vi "Lab Panel V5.20.vi"() -> ()   [LabVIEW 2013] (continued)
                n1788 = property on="O/I  LAB04-1" class="Bool (strict)"("DisabledEnum"=w3333) -> ()  [unwired: 2 in, 2 out]
                n1789 = property on="O/I  LAB04-2" class="Bool (strict)"("DisabledEnum"=w3332) -> ()  [unwired: 2 in, 2 out]
                n1790 = property on="O/I  LAB03-2" class="Bool (strict)"("DisabledEnum"=w3334) -> ()  [unwired: 2 in, 2 out]
                n1791 = Not(x=w3339) -> (.not. x?=w3340:bool)
                n1792 = Not(x=w3338) -> (.not. x?=w3341:bool)
                n1793 = Not(x=w3337) -> (.not. x?=w3342:bool)
                n1794 = property on="RESULT LAB05-2" class="Bool (strict)"("Visible"=w3340) -> ()  [unwired: 2 in, 2 out]
                n1795 = property on="RESULT LAB05-1" class="Bool (strict)"("Visible"=w3341) -> ()  [unwired: 2 in, 2 out]
                n1796 = Not(x=w3336) -> (.not. x?=w3343:bool)
                n1797 = property on="RESULT LAB04-2" class="Bool (strict)"("Visible"=w3342) -> ()  [unwired: 2 in, 2 out]
                n1798 = Not(x=w3335) -> (.not. x?=w3344:bool)
                n1799 = property on="RESULT LAB04-1" class="Bool (strict)"("Visible"=w3343) -> ()  [unwired: 2 in, 2 out]
                n1800 = property on="RESULT LAB03-2" class="Bool (strict)"("Visible"=w3344) -> ()  [unwired: 2 in, 2 out]
              }
              frame #2 {
                # "disable calibrate if any test running"
                n1801 = Or(x=w3367, y=w3366) -> (x .or. y?=w3360:bool)
                n1802 = Or(x=w3369, y=w3368) -> (x .or. y?=w3362:bool)
                n1803 = Or(x=w3373, y=w3372) -> (x .or. y?=w3364:bool)
                n1804 = Or(x=w3371, y=w3370) -> (x .or. y?=w3363:bool)
                n1805 = Or(x=w3375, y=w3374) -> (x .or. y?=w3365:bool)
                n1806 = Or(x=w3363, y=w3362) -> (x .or. y?=w3361:bool)
                n1807 = Or(x=w3365, y=w3364) -> (x .or. y?=w3359:bool)
                n1808 = Or(x=w3361, y=w3360) -> (x .or. y?=w3358:bool)
                n1809 = Or(x=w3359, y=w3358) -> (x .or. y?=w3357:bool)
                n1810 = case shown="False" w3357 {
                  tunnel: [0 2] -> w3356
                  frame False {
                  }
                  frame True {
                  }
                }
                n1811 = property on="JIG TEST" class="Clust (strict)"("DisabledEnum"=w3356) -> ()  [unwired: 2 in, 2 out]
                n1812 = property on="Network Directory" class="Path"("DisabledEnum"=w3356) -> ()  [unwired: 2 in, 2 out]
                n1813 = property on="MAIL SETTINGS" class="Clust (strict)"("DisabledEnum"=w3356) -> ()  [unwired: 2 in, 2 out]
                n1814 = property on="SET (cal)" class="Bool (strict)"("DisabledEnum"=w3356) -> ()  [unwired: 2 in, 2 out]
                n1815 = property on="ADMIN" class="Bool (strict)"("DisabledEnum"=0) -> ()  [unwired: 2 in, 2 out]
              }
            }
          }
          frame #8 {
            # "drive jigs"
            n1816 = stacked-sequence {
              frame #0 {
                # "jig on"
                n1817 = local read "jig cycle"() -> (w3383:dbl)
                n1818 = property on="JIG TEST" class="Clust (strict)"() -> ("DisabledEnum"=w3380:T16)  [unwired: 2 in, 2 out]
                n1819 = Equal?(x=w3380, y=2) -> (x = y?=w3379:bool)
                n1820 = Equal?(x=w3383, y=0) -> (x = y?=w3381:bool)
                n1821 = And(x=w3381, y=w3379) -> (x .and. y?=w3378:bool)
                n1822 = case shown="True" w3378 {
                  frame False {
                  }
                  frame True {
                    n1823 = local read "run lab01-1"() -> (w3394:bool)
                    n1824 = local read "run lab01-2"() -> (w3393:bool)
                    n1825 = local read "run lab02-1"() -> (w3392:bool)
                    n1826 = local read "run lab02-2"() -> (w3391:bool)
                    n1827 = local read "run lab03-1"() -> (w3390:bool)
                    n1828 = local read "run lab03-2"() -> (w3389:bool)
                    n1829 = local read "run lab04-1"() -> (w3388:bool)
                    n1830 = local read "run lab04-2"() -> (w3387:bool)
                    n1831 = local read "run lab05-1"() -> (w3386:bool)
                    n1832 = local read "run lab05-2"() -> (w3385:bool)
                    n1833 = local write "JIG LAB03-2"(w3389) -> ()
                    n1834 = local write "JIG LAB01-1"(w3394) -> ()
                    n1835 = local write "JIG LAB01-2"(w3393) -> ()
                    n1836 = local write "JIG LAB02-1"(w3392) -> ()
                    n1837 = local write "JIG LAB02-2"(w3391) -> ()
                    n1838 = local write "JIG LAB03-1"(w3390) -> ()
                    n1839 = local write "JIG LAB04-1"(w3388) -> ()
                    n1840 = local write "JIG LAB04-2"(w3387) -> ()
                    n1841 = local write "JIG LAB05-1"(w3386) -> ()
                    n1842 = local write "JIG LAB05-2"(w3385) -> ()
                  }
                }
              }
              frame #1 {
                # "jig off"
                n1843 = local read "jig cycle"() -> (w3401:dbl)
                n1844 = local read "on loops"() -> (w3400:dbl)
                n1845 = property on="JIG TEST" class="Clust (strict)"() -> ("DisabledEnum"=w3399:T16)  [unwired: 2 in, 2 out]
                n1846 = Equal?(x=w3399, y=2) -> (x = y?=w3397:bool)
                n1847 = Equal?(x=w3401, y=w3400) -> (x = y?=w3396:bool)
                n1848 = And(x=w3396, y=w3397) -> (x .and. y?=w3395:bool)
                n1849 = case shown="True" w3395 {
                  frame False {
                  }
                  frame True {
                    w3452 = FALSE
                    w3453 = TRUE
                    w3451 = 2
                    n1850 = local read "SELECT LAB05-2"() -> (w3442:T3)
                    n1851 = local read "SELECT LAB04-2"() -> (w3444:T3)
                    n1852 = local read "SELECT LAB04-1"() -> (w3445:T3)
                    n1853 = local read "SELECT LAB05-1"() -> (w3443:T3)
                    n1854 = local read "SELECT LAB03-2"() -> (w3446:T3)
                    n1855 = local read "SELECT LAB02-1"() -> (w3449:T3)
                    n1856 = local read "SELECT LAB03-1"() -> (w3447:T3)
                    n1857 = local read "SELECT LAB02-2"() -> (w3448:T3)
                    n1858 = local read "SELECT LAB01-2"() -> (w3450:T3)
                    n1859 = local read "run lab05-1"() -> (w3412:bool)
                    n1860 = local read "run lab05-2"() -> (w3411:bool)
                    n1861 = local read "run lab04-2"() -> (w3413:bool)
                    n1862 = local read "SELECT LAB01-1"() -> (w3454:T3)
                    n1863 = local read "run lab04-1"() -> (w3414:bool)
                    n1864 = local read "run lab01-1"() -> (w3430:bool)
                    n1865 = local read "run lab01-2"() -> (w3419:bool)
                    n1866 = local read "run lab03-2"() -> (w3415:bool)
                    n1867 = local read "run lab03-1"() -> (w3416:bool)
                    n1868 = local read "run lab02-1"() -> (w3418:bool)
                    n1869 = local read "run lab02-2"() -> (w3417:bool)
                    n1870 = Equal?(x=w3451, y=w3447) -> (x = y?=w3425:bool)
                    n1871 = Equal?(x=w3451, y=w3446) -> (x = y?=w3424:bool)
                    n1872 = Equal?(x=w3451, y=w3445) -> (x = y?=w3423:bool)
                    n1873 = Equal?(x=w3451, y=w3444) -> (x = y?=w3422:bool)
                    n1874 = Equal?(x=w3451, y=w3443) -> (x = y?=w3421:bool)
                    n1875 = Equal?(x=w3451, y=w3442) -> (x = y?=w3420:bool)
                    n1876 = Equal?(x=w3451, y=w3454) -> (x = y?=w3431:bool)
                    n1877 = Equal?(x=w3451, y=w3449) -> (x = y?=w3427:bool)
                    n1878 = Equal?(x=w3451, y=w3448) -> (x = y?=w3426:bool)
                    n1879 = Equal?(x=w3451, y=w3450) -> (x = y?=w3428:bool)
                    n1880 = And(x=w3422, y=w3413) -> (x .and. y?=w3404:bool)
                    n1881 = And(x=w3425, y=w3416) -> (x .and. y?=w3407:bool)
                    n1882 = And(x=w3423, y=w3414) -> (x .and. y?=w3405:bool)
                    n1883 = And(x=w3420, y=w3411) -> (x .and. y?=w3402:bool)
                    n1884 = And(x=w3426, y=w3417) -> (x .and. y?=w3408:bool)
                    n1885 = And(x=w3424, y=w3415) -> (x .and. y?=w3406:bool)
                    n1886 = And(x=w3421, y=w3412) -> (x .and. y?=w3403:bool)
                    n1887 = And(x=w3428, y=w3419) -> (x .and. y?=w3410:bool)
                    n1888 = And(x=w3431, y=w3430) -> (x .and. y?=w3429:bool)
                    n1889 = And(x=w3427, y=w3418) -> (x .and. y?=w3409:bool)
                    n1890 = Select(t=w3453, s=w3429, f=w3452) -> (s? t:f=w3432:bool)
                    n1891 = Select(t=w3453, s=w3410, f=w3452) -> (s? t:f=w3433:bool)
                    n1892 = Select(t=w3453, s=w3409, f=w3452) -> (s? t:f=w3434:bool)
                    n1893 = Select(t=w3453, s=w3408, f=w3452) -> (s? t:f=w3435:bool)
                    n1894 = Select(t=w3453, s=w3407, f=w3452) -> (s? t:f=w3436:bool)
                    n1895 = Select(t=w3453, s=w3406, f=w3452) -> (s? t:f=w3437:bool)
                    n1896 = Select(t=w3453, s=w3405, f=w3452) -> (s? t:f=w3438:bool)
                    n1897 = Select(t=w3453, s=w3404, f=w3452) -> (s? t:f=w3439:bool)
                    n1898 = Select(t=w3453, s=w3403, f=w3452) -> (s? t:f=w3440:bool)
                    n1899 = Select(t=w3453, s=w3402, f=w3452) -> (s? t:f=w3441:bool)
                    n1900 = local write "JIG LAB03-2"(w3437) -> ()
                    n1901 = local write "JIG LAB02-1"(w3434) -> ()
                    n1902 = local write "JIG LAB02-2"(w3435) -> ()
                    n1903 = local write "JIG LAB01-2"(w3433) -> ()
                    n1904 = local write "JIG LAB03-1"(w3436) -> ()
                    n1905 = local write "JIG LAB01-1"(w3432) -> ()
                    n1906 = local write "JIG LAB05-2"(w3441) -> ()
                    n1907 = local write "JIG LAB04-1"(w3438) -> ()
                    n1908 = local write "JIG LAB05-1"(w3440) -> ()
                    n1909 = local write "JIG LAB04-2"(w3439) -> ()
                  }
                }
              }
            }
          }
          frame #9 {
            # "enable  jig test output if no test busy"
            n1910 = property on="JIG TEST" class="Clust (strict)"() -> ("DisabledEnum"=w3457:T16)  [unwired: 2 in, 2 out]
            n1911 = Equal?(x=w3457, y=0) -> (x = y?=w3455:bool)
            n1912 = case shown="True" w3455 {
              frame False {
              }
              frame True {
                n1913 = local read "JIG TEST"() -> (w3468:T10)
                n1914 = Unbundle(w3468) -> ("LAB01-1"=w3467:bool, "LAB01-2"=w3466:bool, "LAB02-1"=w3465:bool, "LAB02-2"=w3464:bool, "LAB03-1"=w3463:bool, "LAB03-2"=w3462:bool, "LAB04-1"=w3461:bool, "LAB04-2"=w3460:bool, "LAB05-1"=w3459:bool, "LAB05-2"=w3458:bool)
                n1915 = local write "JIG LAB05-1"(w3459) -> ()
                n1916 = local write "JIG LAB05-2"(w3458) -> ()
                n1917 = local write "JIG LAB04-1"(w3461) -> ()
                n1918 = local write "JIG LAB04-2"(w3460) -> ()
                n1919 = local write "JIG LAB03-2"(w3462) -> ()
                n1920 = local write "JIG LAB01-1"(w3467) -> ()
                n1921 = local write "JIG LAB02-1"(w3465) -> ()
                n1922 = local write "JIG LAB03-1"(w3463) -> ()
                n1923 = local write "JIG LAB01-2"(w3466) -> ()
                n1924 = local write "JIG LAB02-2"(w3464) -> ()
              }
            }
          }
          frame #10 {
            # "Drive digital output and reset USB and temperature network if required."
            n1925 = global read "Global display 3.vi" "cycle O/F"() -> (w3478:bool)
            n1926 = local read "O/I  LAB05-2"() -> (w3471:bool)
            n1927 = local read "O/I  LAB05-1"() -> (w3473:bool)
            n1928 = local read "JIG LAB05-2"() -> (w3470:bool)
            n1929 = local read "O/I  LAB04-2"() -> (w3475:bool)
            n1930 = local read "JIG LAB05-1"() -> (w3472:bool)
            n1931 = local read "JIG LAB04-2"() -> (w3474:bool)
            n1932 = local read "O/I  LAB03-1"() -> (w3489:bool)
            n1933 = local read "O/I  LAB04-1"() -> (w3485:bool)
            n1934 = local read "O/I  LAB02-1"() -> (w3493:bool)
            n1935 = local read "O/I  LAB02-2"() -> (w3491:bool)
            n1936 = local read "O/I  LAB03-2"() -> (w3487:bool)
            n1937 = local read "JIG LAB04-1"() -> (w3484:bool)
            n1938 = local read "JIG LAB03-2"() -> (w3486:bool)
            n1939 = local read "O/I  LAB01-2"() -> (w3495:bool)
            n1940 = local read "JIG LAB02-1"() -> (w3492:bool)
            n1941 = local read "JIG LAB02-2"() -> (w3490:bool)
            n1942 = local read "JIG LAB03-1"() -> (w3488:bool)
            n1943 = local read "O/I  LAB01-1"() -> (w3497:bool)
            n1944 = local read "JIG LAB01-2"() -> (w3494:bool)
            n1945 = local read "JIG LAB01-1"() -> (w3496:bool)
            n1946 = case shown="False" w3478 {
              tunnel: [w3578 FALSE] -> w3477
              frame False {
                n1947 = local read "Analog error"() -> (w3577:bool)
                n1948 = local read "Reset Measuring"() -> (w3576:bool)
                n1949 = Or(x=w3576, y=w3577) -> (x .or. y?=w3578:bool)
              }
              frame True {
              }
            }
            n1950 = Build Array(w3490, w3489, w3488, w3487, w3486, w3485, w3484) -> (w3482:bool[])
            n1951 = Build Array(w3497, w3496, w3495, w3494, w3493, w3492, w3491) -> (w3483:bool[])
            n1952 = Build Array(w3475, w3474, w3473, w3472, w3471, w3470, FALSE) -> (w3481:bool[])
            n1953 = Not(x=w3478) -> (.not. x?=w3479:bool)
            n1954 = local read "Simulate"() -> (w3480:bool)
            n1955 = And(x=w3479, y=w3477) -> (x .and. y?=w3476:bool)
            n1956 = stacked-sequence {
              tunnel: w3483 -> [w3501 w3507]
              tunnel: w3482 -> [w3500 w3506]
              tunnel: w3481 -> [w3499 w3505]
              tunnel: w3480 -> [w3498 w3508]
              tunnel: w3476 -> [_ w3509]
              frame #0 {
                # "drive outputs for normal use"
                n1957 = case shown="False" w3498 {
                  tunnel: w3501 -> [w3504 _]
                  tunnel: w3500 -> [w3503 _]
                  tunnel: w3499 -> [w3502 _]
                  frame False {
                    n1958 = call "sub vi - Drive Relays All v6.vi"("Array #2"=w3502, "Array #1"=w3503, "Array #0"=w3504) -> ()  [unwired: 8 in, 1 out]
                  }
                  frame True {
                  }
                }
              }
              frame #1 {
                # "system reset routine"
                n1959 = case shown="True" w3509 {
                  tunnel: w3508 -> [_ w3513]
                  tunnel: w3507 -> [_ w3512]
                  tunnel: w3506 -> [_ w3511]
                  tunnel: w3505 -> [_ w3510]
                  frame False {
                  }
                  frame True {
                    n1960 = stacked-sequence {
                      seq-local: [w3515 _ _] -> [_ w3521 _]
                      tunnel: w3513 -> [_ w3525 _]
                      tunnel: w3512 -> [_ w3524 _]
                      tunnel: w3511 -> [_ w3523 _]
                      tunnel: w3510 -> [_ w3522 _]
                      frame #0 {
                        n1961 = case shown="False" "Auto Reset" {
                          tunnel: [w3518 FALSE] -> w3516
                          frame False {
                            n1962 = Two Button Dialog(message="System reset") -> (T button?=w3518:bool)  [unwired: 2 in]
                          }
                          frame True {
                          }
                        }
                        n1963 = local write "Tab Control 2"(5) -> ()
                        n1964 = Or(x="Auto Reset", y=w3516) -> (x .or. y?=w3515:bool)
                      }
                      frame #1 {
                        n1965 = case shown="True" w3521 {
                          tunnel: w3525 -> [_ w3531]
                          tunnel: w3524 -> [_ w3530]
                          tunnel: w3523 -> [_ w3529]
                          tunnel: w3522 -> [_ w3528]
                          frame False {
                          }
                          frame True {
                            n1966 = stacked-sequence {
                              tunnel: w3531 -> [_ w3549 _]
                              tunnel: bool[] [] -> [w3534 w3548 w3557]
                              tunnel: w3530 -> [_ _ w3556]
                              tunnel: w3529 -> [w3533 _ w3555]
                              tunnel: w3528 -> [w3532 _ w3554]
                              tunnel: 3000 -> [w3535 _ w3553]
                              frame #0 {
                                # "switch off test stations for system reset"
                                n1967 = stacked-sequence {
                                tunnel: w3535 -> [w3539 w3543 w3545]
                                tunnel: w3534 -> [w3538 w3542 w3546]
                                tunnel: w3533 -> [w3537 _ _]
                                tunnel: w3532 -> [w3536 w3541 _]
                                frame #0 {
                                # "drive 1st 7 inputs"
                                n1968 = call "sub vi - Drive Relays All v6.vi"("Array #2"=w3536, "Array #1"=w3537, "Array #0"=w3538) -> ()  [unwired: 8 in, 1 out]
                                n1969 = call "Message Display V1.vi"("Message"="Delay off LAB 01-1 to 02-1", "Delay mS"=w3539) -> ()  [unwired: 10 in]
                                }
                                frame #1 {
                                # "drive 2nd 7 inputs"
                                n1970 = call "sub vi - Drive Relays All v6.vi"("Array #2"=w3541, "Array #1"=w3542, "Array #0"=w3542) -> ()  [unwired: 8 in, 1 out]
                                n1971 = call "Message Display V1.vi"("Message"="Delay off LAB 02-2 to 04-1", "Delay mS"=w3543) -> ()  [unwired: 10 in]
                                }
                                frame #2 {
                                # "drive 3rd 7 inputs"
                                n1972 = call "sub vi - Drive Relays All v6.vi"("Array #2"=w3546, "Array #1"=w3546, "Array #0"=w3546) -> ()  [unwired: 8 in, 1 out]
                                n1973 = call "Message Display V1.vi"("Message"="Delay off LAB 04-2 to 05-2", "Delay mS"=w3545) -> ()  [unwired: 10 in]
                                }
                                }
                              }
                              frame #1 {
                                # "reset all usb modules"
                                n1974 = stacked-sequence {
                                tunnel: w3549 -> [_ w3552]
                                tunnel: w3548 -> [w3551 _]
                                frame #0 {
                                n1975 = call "sub vi - Drive Relays All v6.vi"("Array #2"=bool[] [FALSE, FALSE, FALSE, FALSE, FALSE, FALSE, TRUE], "Array #1"=w3551, "Array #0"=w3551) -> ()  [unwired: 8 in, 1 out]
                                }
                                frame #1 {
                                n1976 = call "Reset Meas v 4.vi"("simulate"=w3552) -> ()  [unwired: 11 in]
                                }
                                }
                              }
                              frame #2 {
                                # "switch test stations back on after reset"
                                n1977 = stacked-sequence {
                                tunnel: w3557 -> [w3561 w3564 _]
                                tunnel: w3556 -> [w3560 w3566 w3571]
                                tunnel: w3553 -> [w3559 w3562 w3568]
                                tunnel: w3555 -> [_ w3565 w3570]
                                tunnel: w3554 -> [_ _ w3567]
                                frame #0 {
                                # "drive 1st 7 inputs"
                                n1978 = call "sub vi - Drive Relays All v6.vi"("Array #2"=w3561, "Array #1"=w3561, "Array #0"=w3560) -> ()  [unwired: 8 in, 1 out]
                                n1979 = call "Message Display V1.vi"("Message"="Delay on LAB 01-1 to 02-1", "Delay mS"=w3559) -> ()  [unwired: 10 in]
                                }
                                frame #1 {
                                # "drive 1st & 2nd outputs"
                                n1980 = call "sub vi - Drive Relays All v6.vi"("Array #2"=w3564, "Array #1"=w3565, "Array #0"=w3566) -> ()  [unwired: 8 in, 1 out]
                                n1981 = call "Message Display V1.vi"("Message"="Delay on LAB 02-2 to 04-1", "Delay mS"=w3562) -> ()  [unwired: 10 in]
                                }
                                frame #2 {
                                n1982 = call "sub vi - Drive Relays All v6.vi"("Array #2"=w3567, "Array #1"=w3570, "Array #0"=w3571) -> ()  [unwired: 8 in, 1 out]
                                n1983 = call "Message Display V1.vi"("Message"="Delay on LAB 04-2 to 05-2", "Delay mS"=w3568) -> ()  [unwired: 10 in]
                                }
                                }
                              }
                            }
                          }
                        }
                      }
                      frame #2 {
                        w3574 = 0
                        w3575 = FALSE
                        # "set all back to zero"
                        n1984 = local read "Resets Done"() -> (w3573:dbl)
                        n1985 = local write "Reset Measuring"(w3575) -> ()
                        n1986 = local write "Analog error"(w3575) -> ()
                        n1987 = local write "Error USB #0"(w3575) -> ()
                        n1988 = local write "Error USB #1"(w3575) -> ()
                        n1989 = local write "Error USB #2"(w3575) -> ()
                        n1990 = local write "Er USB#0"(w3574) -> ()
                        n1991 = local write "Er USB#1"(w3574) -> ()
                        n1992 = local write "Er USB#2"(w3574) -> ()
                        n1993 = Increment(x=w3573) -> (x+1=→"Resets Done":dbl)
                      }
                    }
                  }
                }
              }
            }
          }
          frame #11 {
            # "get all analog values from USB devices"
            n1994 = local read "on loops"() -> (w3586:dbl)
            n1995 = local read "jig cycle"() -> (w3583:dbl)
            n1996 = Add(x=w3586, y=1) -> (x+y=w3584:dbl)
            n1997 = Equal?(x=w3583, y=1) -> (x = y?=w3580:bool)
            n1998 = Equal?(x=w3583, y=w3584) -> (x = y?=w3582:bool)
            n1999 = Or(x=w3580, y=w3582) -> (x .or. y?=w3581:bool)
            n2000 = global write "Global display 3.vi" "cycle O/F"(w3580) -> ()
            n2001 = case shown="True" w3581 {
              tunnel: w3580 -> [_ w3590]
              frame False {
              }
              frame True {
                n2002 = local read "Simulate"() -> (w3593:bool)
                n2003 = case shown="False" w3593 {
                  tunnel: [w3609 0.3 ("Analog loop time")] -> w3600
                  tunnel: [w3608 dynamicdata[] [] ("array GRAPH")] -> w3599
                  tunnel: [w3607 w3614] -> w3598
                  tunnel: [w3606 w3614] -> w3597
                  tunnel: [w3605 w3614] -> w3596
                  tunnel: [w3604 w3614] -> w3595
                  tunnel: [w3603 w3614] -> w3594
                  tunnel: w3590 -> [_ w3618]
                  tunnel: [w3602 "Ambient Volts"] -> w3589
                  tunnel: [w3601 bool[] []] -> w3588
                  frame False {
                    n2004 = call "sub vi - Read Analog All v9.3.vi"() -> ("Analog loop time"=w3609:dbl, "array GRAPH"=w3608:dynamicdata[], "LAB01"=w3607:T26, "LAB02"=w3606:T27, "LAB03"=w3605:T28, "LAB04"=w3604:T29, "deg C"=w3602:dbl, "USB Error"=w3601:bool[], "LAB05"=w3603:T30)  [unwired: 7 in]
                  }
                  frame True {
                    n2005 = local read "ON amps"() -> (w3612:dbl)
                    n2006 = local read "OFF amps"() -> (w3613:dbl)
                    n2007 = local read "VOLTS"() -> (w3616:dbl)
                    n2008 = local read "PF"() -> (w3615:dbl)
                    n2009 = Select(t=w3612, s=w3618, f=w3613) -> (s? t:f=w3617:dbl)
                    n2010 = Bundle("OFF amps"=w3617, "VOLTS"=w3616, "PF"=w3615, "OFF amps"=w3617, "VOLTS"=w3616, "PF"=w3615) -> (w3614:T31)  [unwired: 1 in]
                  }
                }
                n2011 = local read "Simulate"() -> (w3592:bool)
                n2012 = stacked-sequence {
                  seq-local: [w3623 _ _ _ _ _ _ _] -> [_ _ _ _ _ _ _ _]
                  seq-local: [w3622 _ _ _ _ _ _ _] -> [_ _ _ _ _ _ _ _]
                  seq-local: [w3621 _ _ _ _ _ _ _] -> [_ _ _ _ _ _ _ w3818]
                  tunnel: w3600 -> [_ w3676 _ _ _ _ _ _]
                  tunnel: w3599 -> [_ w3673 _ _ _ _ _ _]
                  tunnel: w3598 -> [_ _ w3703 _ _ _ _ _]
                  tunnel: w3597 -> [_ _ _ w3731 _ _ _ _]
                  tunnel: w3596 -> [_ _ _ _ w3759 _ _ _]
                  tunnel: w3595 -> [_ _ _ _ _ w3787 _ _]
                  tunnel: w3594 -> [_ _ _ _ _ _ w3815 _]
                  tunnel: w3592 -> [_ _ w3702 w3730 w3758 w3786 w3814 w3820]
                  tunnel: T14 {"1  (A) cal"=1.0, "1 (V) cal"=1.0, "1 (PF) cal"=1.0, "1 (TL) cal"=1.0, "1 (TN) cal"=1.0, "2 (A) cal"=1.0, "2 (V) cal"=1.0, "2 (PF) cal"=1.0, "2 (TL) cal"=1.0, "2 (TN) cal"=1.0} ("CAL LAB01") -> [_ _ w3701 w3729 w3757 w3785 w3813 _]
                  tunnel: w3589 -> [_ _ _ _ _ _ _ w3819]
                  tunnel: w3588 -> [w3626 _ _ _ _ _ _ _]
                  frame #0 {
                    n2013 = Index Array(array=w3626, index=2) -> (element=w3621:bool)
                    n2014 = Index Array(array=w3626, index=1) -> (element=w3622:bool)
                    n2015 = Index Array(array=w3626, index=0) -> (element=w3623:bool)
                    n2016 = local write "Error USB #2"(w3621) -> ()
                    n2017 = local write "Error USB #0"(w3623) -> ()
                    n2018 = local write "Error USB #1"(w3622) -> ()
                    n2019 = stacked-sequence {
                      tunnel: w3623 -> [w3630 _ _ _]
                      tunnel: w3622 -> [_ w3635 _ _]
                      tunnel: 0 -> [w3629 w3634 w3639 _]
                      tunnel: w3621 -> [_ _ w3640 _]
                      frame #0 {
                        n2020 = case shown="True" w3630 {
                          tunnel: w3629 -> [w3631 _]
                          frame False {
                            n2021 = local write "Er USB#0"(w3631) -> ()
                          }
                          frame True {
                            n2022 = local read "Er USB#0"() -> (w3633:dbl)
                            n2023 = Increment(x=w3633) -> (x+1=→"Er USB#0":dbl)
                          }
                        }
                      }
                      frame #1 {
                        n2024 = case shown="True" w3635 {
                          tunnel: w3634 -> [w3636 _]
                          frame False {
                            n2025 = local write "Er USB#1"(w3636) -> ()
                          }
                          frame True {
                            n2026 = local read "Er USB#1"() -> (w3638:dbl)
                            n2027 = Increment(x=w3638) -> (x+1=→"Er USB#1":dbl)
                          }
                        }
                      }
                      frame #2 {
                        n2028 = case shown="True" w3640 {
                          tunnel: w3639 -> [w3641 _]
                          frame False {
                            n2029 = local write "Er USB#2"(w3641) -> ()
                          }
                          frame True {
                            n2030 = local read "Er USB#2"() -> (w3643:dbl)
                            n2031 = Increment(x=w3643) -> (x+1=→"Er USB#2":dbl)
                          }
                        }
                      }
                      frame #3 {
                        w3649 = 5
                        n2032 = local read "Er USB#2"() -> (w3650:dbl)
                        n2033 = local read "Er USB#0"() -> (w3652:dbl)
                        n2034 = local read "Er USB#1"() -> (w3651:dbl)
                        n2035 = Greater Or Equal?(x=w3652, y=w3649) -> (x >= y?=w3647:bool)
                        n2036 = Greater Or Equal?(x=w3651, y=w3649) -> (x >= y?=w3646:bool)
                        n2037 = Greater Or Equal?(x=w3650, y=w3649) -> (x >= y?=w3645:bool)
                        n2038 = Or(x=w3647, y=w3646) -> (x .or. y?=w3648:bool)
                        n2039 = Or(x=w3648, y=w3645) -> (x .or. y?=→"Analog error":bool)
                      }
                    }
                  }
                  frame #1 {
                    # "display graph data on ADM page"
                    n2040 = local write "AI"(TRUE) -> ()
                    n2041 = global write "Global 1.vi" "RATE(Hz)"("RATE (Hz)") -> ()
                    n2042 = global write "Global 1.vi" "SAMPLES"("SAMPLES") -> ()
                    n2043 = Index Array(array=w3673, index=6) -> (element=→"LAB04-1 (GRAPH)":dynamicdata)
                    n2044 = Index Array(array=w3673, index=7) -> (element=→"LAB04-2 (GRAPH)":dynamicdata)
                    n2045 = Index Array(array=w3673, index=9) -> (element=→"LAB05-2 (GRAPH)":dynamicdata)
                    n2046 = Index Array(array=w3673, index=8) -> (element=→"LAB05-1 (GRAPH)":dynamicdata)
                    n2047 = Index Array(array=w3673, index=5) -> (element=→"LAB03-2 (GRAPH)":dynamicdata)
                    n2048 = Index Array(array=w3673, index=0) -> (element=→"LAB01-1 (GRAPH)":dynamicdata)
                    n2049 = Index Array(array=w3673, index=1) -> (element=→"LAB01-2 (GRAPH)":dynamicdata)
                    n2050 = Index Array(array=w3673, index=2) -> (element=→"LAB02-1 (GRAPH)":dynamicdata)
                    n2051 = Index Array(array=w3673, index=3) -> (element=→"LAB02-2 (GRAPH)":dynamicdata)
                    n2052 = Index Array(array=w3673, index=4) -> (element=→"LAB03-1 (GRAPH)":dynamicdata)
                    "AI loop time" <- w3676
                  }
                  frame #2 {
                    n2053 = case shown="False" w3702 {
                      tunnel: [w3704 w3705] -> w3700
                      tunnel: w3701 -> [_ w3705]
                      frame False {
                        n2054 = local read "CAL LAB01"() -> (w3704:T14)
                      }
                      frame True {
                      }
                    }
                    n2055 = Unbundle By Name(w3703) -> ("OFF amps"=w3699:dbl, "VOLTS"=w3698:dbl, "PF"=w3697:dbl, "OFF amps"=w3696:dbl, "VOLTS"=w3695:dbl, "PF"=w3694:dbl)
                    n2056 = Unbundle By Name(w3700) -> ("1  (A) cal"=w3693:dbl, "1 (V) cal"=w3692:dbl, "1 (PF) cal"=w3691:dbl, "2 (A) cal"=w3690:dbl, "2 (V) cal"=w3689:dbl, "2 (PF) cal"=w3688:dbl)  [unwired: 4 out]
                    n2057 = Multiply(x=w3699, y=w3693) -> (x*y=w3686:dbl)
                    n2058 = Multiply(x=w3698, y=w3692) -> (x*y=w3685:dbl)
                    n2059 = Multiply(x=w3697, y=w3691) -> (x*y=w3684:dbl)
                    n2060 = Multiply(x=w3696, y=w3690) -> (x*y=w3682:dbl)
                    n2061 = Multiply(x=w3695, y=w3689) -> (x*y=w3681:dbl)
                    n2062 = Multiply(x=w3694, y=w3688) -> (x*y=w3680:dbl)
                    n2063 = local read "SIG LAB01-1"() -> (w3687:T2)
                    n2064 = local read "SIG LAB01-2"() -> (w3683:T2)
                    n2065 = Bundle By Name(cluster=w3687, "AMPS"=w3686, "VOLTS"=w3685, "PF"=w3684) -> (w3679:T2)
                    n2066 = Bundle By Name(cluster=w3683, "AMPS"=w3682, "VOLTS"=w3681, "PF"=w3680) -> (w3678:T2)
                    n2067 = global write "Global display 1.vi" "SIG LAB01-2"(w3678) -> ()
                    n2068 = global write "Global display 1.vi" "SIG LAB01-1"(w3679) -> ()
                    n2069 = local write "SIG LAB01-2"(w3678) -> ()
                    n2070 = local write "SIG LAB01-1"(w3679) -> ()
                  }
                  frame #3 {
                    n2071 = Unbundle By Name(w3731) -> ("OFF amps"=w3727:dbl, "VOLTS"=w3726:dbl, "PF"=w3725:dbl, "OFF amps"=w3724:dbl, "VOLTS"=w3723:dbl, "PF"=w3722:dbl)
                    n2072 = case shown="True" w3730 {
                      tunnel: [w3732 w3733] -> w3728
                      tunnel: w3729 -> [_ w3733]
                      frame False {
                        n2073 = local read "CAL LAB02"() -> (w3732:T15)
                      }
                      frame True {
                      }
                    }
                    n2074 = Unbundle By Name(w3728) -> ("1  (A) cal"=w3721:dbl, "1 (V) cal"=w3720:dbl, "1 (PF) cal"=w3719:dbl, "2 (A) cal"=w3718:dbl, "2 (V) cal"=w3717:dbl, "2 (PF) cal"=w3716:dbl)  [unwired: 4 out]
                    n2075 = Multiply(x=w3727, y=w3721) -> (x*y=w3714:dbl)
                    n2076 = Multiply(x=w3726, y=w3720) -> (x*y=w3713:dbl)
                    n2077 = Multiply(x=w3725, y=w3719) -> (x*y=w3712:dbl)
                    n2078 = Multiply(x=w3724, y=w3718) -> (x*y=w3710:dbl)
                    n2079 = Multiply(x=w3723, y=w3717) -> (x*y=w3709:dbl)
                    n2080 = Multiply(x=w3722, y=w3716) -> (x*y=w3708:dbl)
                    n2081 = local read "SIG LAB02-1"() -> (w3715:T2)
                    n2082 = local read "SIG LAB02-2"() -> (w3711:T2)
                    n2083 = Bundle By Name(cluster=w3715, "AMPS"=w3714, "VOLTS"=w3713, "PF"=w3712) -> (w3707:T2)
                    n2084 = Bundle By Name(cluster=w3711, "AMPS"=w3710, "VOLTS"=w3709, "PF"=w3708) -> (w3706:T2)
                    n2085 = global write "Global display 1.vi" "SIG LAB02-1"(w3707) -> ()
                    n2086 = local write "SIG LAB02-2"(w3706) -> ()
                    n2087 = global write "Global display 1.vi" "SIG LAB02-2"(w3706) -> ()
                    n2088 = local write "SIG LAB02-1"(w3707) -> ()
                  }
                  frame #4 {
                    n2089 = Unbundle By Name(w3759) -> ("OFF amps"=w3755:dbl, "VOLTS"=w3754:dbl, "PF"=w3753:dbl, "OFF amps"=w3752:dbl, "VOLTS"=w3751:dbl, "PF"=w3750:dbl)
                    n2090 = case shown="True" w3758 {
                      tunnel: [w3760 w3761] -> w3756
                      tunnel: w3757 -> [_ w3761]
                      frame False {
                        n2091 = local read "CAL LAB03"() -> (w3760:T14)
                      }
                      frame True {
                      }
                    }
                    n2092 = Unbundle By Name(w3756) -> ("1  (A) cal"=w3749:dbl, "1 (V) cal"=w3748:dbl, "1 (PF) cal"=w3747:dbl, "2 (A) cal"=w3746:dbl, "2 (V) cal"=w3745:dbl, "2 (PF) cal"=w3744:dbl)  [unwired: 4 out]
                    n2093 = Multiply(x=w3755, y=w3749) -> (x*y=w3742:dbl)
                    n2094 = Multiply(x=w3754, y=w3748) -> (x*y=w3736:dbl)
                    n2095 = Multiply(x=w3753, y=w3747) -> (x*y=w3741:dbl)
                    n2096 = Multiply(x=w3752, y=w3746) -> (x*y=w3739:dbl)
                    n2097 = Multiply(x=w3751, y=w3745) -> (x*y=w3738:dbl)
                    n2098 = Multiply(x=w3750, y=w3744) -> (x*y=w3737:dbl)
                    n2099 = local read "SIG LAB03-1"() -> (w3743:T2)
                    n2100 = local read "SIG LAB03-2"() -> (w3740:T2)
                    n2101 = Bundle By Name(cluster=w3743, "AMPS"=w3742, "VOLTS"=w3736, "PF"=w3741) -> (w3735:T2)
                    n2102 = Bundle By Name(cluster=w3740, "AMPS"=w3739, "VOLTS"=w3738, "PF"=w3737) -> (w3734:T2)
                    n2103 = global write "Global display 1.vi" "SIG LAB03-1"(w3735) -> ()
                    n2104 = global write "Global display 1.vi" "SIG LAB03-2"(w3734) -> ()
                    n2105 = local write "SIG LAB03-2"(w3734) -> ()
                    n2106 = local write "SIG LAB03-1"(w3735) -> ()
                  }
                  frame #5 {
                    n2107 = case shown="False" w3786 {
                      tunnel: [w3788 w3789] -> w3784
                      tunnel: w3785 -> [_ w3789]
                      frame False {
                        n2108 = local read "CAL LAB04"() -> (w3788:T14)
                      }
                      frame True {
                      }
                    }
                    n2109 = Unbundle By Name(w3787) -> ("OFF amps"=w3783:dbl, "VOLTS"=w3782:dbl, "PF"=w3781:dbl, "OFF amps"=w3780:dbl, "VOLTS"=w3779:dbl, "PF"=w3778:dbl)
                    n2110 = Unbundle By Name(w3784) -> ("1  (A) cal"=w3777:dbl, "1 (V) cal"=w3776:dbl, "1 (PF) cal"=w3775:dbl, "2 (A) cal"=w3774:dbl, "2 (V) cal"=w3773:dbl, "2 (PF) cal"=w3772:dbl)  [unwired: 4 out]
                    n2111 = Multiply(x=w3783, y=w3777) -> (x*y=w3770:dbl)
                    n2112 = Multiply(x=w3782, y=w3776) -> (x*y=w3769:dbl)
                    n2113 = Multiply(x=w3781, y=w3775) -> (x*y=w3768:dbl)
                    n2114 = Multiply(x=w3780, y=w3774) -> (x*y=w3766:dbl)
                    n2115 = Multiply(x=w3779, y=w3773) -> (x*y=w3765:dbl)
                    n2116 = Multiply(x=w3778, y=w3772) -> (x*y=w3764:dbl)
                    n2117 = local read "SIG LAB04-1"() -> (w3771:T2)
                    n2118 = local read "SIG LAB04-2"() -> (w3767:T2)
                    n2119 = Bundle By Name(cluster=w3771, "AMPS"=w3770, "VOLTS"=w3769, "PF"=w3768) -> (w3763:T2)
                    n2120 = Bundle By Name(cluster=w3767, "AMPS"=w3766, "VOLTS"=w3765, "PF"=w3764) -> (w3762:T2)
                    n2121 = global write "Global display 1.vi" "SIG LAB04-2"(w3762) -> ()
                    n2122 = global write "Global display 1.vi" "SIG LAB04-1"(w3763) -> ()
                    n2123 = local write "SIG LAB04-2"(w3762) -> ()
                    n2124 = local write "SIG LAB04-1"(w3763) -> ()
                  }
                  frame #6 {
                    n2125 = Unbundle By Name(w3815) -> ("OFF amps"=w3811:dbl, "VOLTS"=w3792:dbl, "PF"=w3810:dbl, "OFF amps"=w3809:dbl, "VOLTS"=w3808:dbl, "PF"=w3807:dbl)
                    n2126 = case shown="False" w3814 {
                      tunnel: [w3816 w3817] -> w3812
                      tunnel: w3813 -> [_ w3817]
                      frame False {
                        n2127 = local read "CAL LAB05"() -> (w3816:T14)
                      }
                      frame True {
                      }
                    }
                    n2128 = Unbundle By Name(w3812) -> ("1  (A) cal"=w3806:dbl, "1 (V) cal"=w3805:dbl, "1 (PF) cal"=w3804:dbl, "2 (A) cal"=w3803:dbl, "2 (V) cal"=w3802:dbl, "2 (PF) cal"=w3801:dbl)  [unwired: 4 out]
                    n2129 = Multiply(x=w3811, y=w3806) -> (x*y=w3799:dbl)
                    n2130 = Multiply(x=w3792, y=w3805) -> (x*y=w3798:dbl)
                    n2131 = Multiply(x=w3810, y=w3804) -> (x*y=w3797:dbl)
                    n2132 = Multiply(x=w3809, y=w3803) -> (x*y=w3795:dbl)
                    n2133 = Multiply(x=w3808, y=w3802) -> (x*y=w3794:dbl)
                    n2134 = Multiply(x=w3807, y=w3801) -> (x*y=w3793:dbl)
                    n2135 = local read "SIG LAB05-1"() -> (w3800:T2)
                    n2136 = local read "SIG LAB05-2"() -> (w3796:T2)
                    n2137 = Bundle By Name(cluster=w3800, "AMPS"=w3799, "VOLTS"=w3798, "PF"=w3797) -> (w3791:T2)
                    n2138 = Bundle By Name(cluster=w3796, "AMPS"=w3795, "VOLTS"=w3794, "PF"=w3793) -> (w3790:T2)
                    n2139 = global write "Global display 1.vi" "SIG LAB05-1"(w3791) -> ()
                    n2140 = global write "Global display 1.vi" "SIG LAB05-2"(w3790) -> ()
                    n2141 = local write "SIG LAB05-2"(w3790) -> ()
                    n2142 = local write "SIG LAB05-1"(w3791) -> ()
                  }
                  frame #7 {
                    n2143 = case shown="False" w3818 {
                      tunnel: w3820 -> [w3822 _]
                      tunnel: w3819 -> [w3821 _]
                      frame False {
                        # "update ambient referance temperature"
                        n2144 = case shown="True" w3822 {
                          tunnel: [w3825 100.0] -> w3824
                          frame False {
                            n2145 = local read "TEMP REF cal"() -> (w3825:dbl)
                          }
                          frame True {
                          }
                        }
                        n2146 = local read "Panel #"() -> (w3823:dbl)
                        n2147 = case shown="1" w3823 {
                          tunnel: w3824 -> [_ w3831]
                          tunnel: w3821 -> [_ w3830]
                          frame 0, Default {
                          }
                          frame 1 {
                            n2148 = Multiply(x=w3831, y=w3830) -> (x*y=w3829:dbl)
                            n2149 = Subtract(x=w3829, y=272) -> (x-y=w3827:dbl)
                            "Amb Tp" <- w3827
                            n2150 = local write "Ref deg C"(w3827) -> ()
                          }
                        }
                        "deg C (volts)" <- w3821
                      }
                      frame True {
                      }
                    }
                  }
                }
              }
            }
          }
          frame #12 {
            # "save test data to file"
            n2151 = Get Date/Time In Seconds() -> (seconds since 1Jan1904=w3832:timestamp)
            "File Time Stamp" <- w3832
            n2152 = local read "on loops"() -> (w3851:dbl)
            n2153 = local read "jig cycle"() -> (w3848:dbl)
            n2154 = Format Date/Time String(time format string (%c)="%H:%M%:%S", seconds (now)=w3832) -> (date/time string=w3836:string)  [unwired: 1 in]
            n2155 = Add(x=w3851, y=2) -> (x+y=w3849:dbl)
            n2156 = Build Array(w3836) -> (w3835:string[])
            n2157 = Equal?(x=w3848, y=1) -> (x = y?=w3834:bool)
            n2158 = Equal?(x=w3848, y=w3849) -> (x = y?=w3833:bool)
            n2159 = stacked-sequence {
              tunnel: w3847 -> [w3857 _ _ _ _ _ _ _ _ _]
              tunnel: w3846 -> [_ w3933 _ _ _ _ _ _ _ _]
              tunnel: w3845 -> [_ _ w4013 _ _ _ _ _ _ _]
              tunnel: w3844 -> [_ _ _ w4093 _ _ _ _ _ _]
              tunnel: w3843 -> [_ _ _ _ w4173 _ _ _ _ _]
              tunnel: w3842 -> [_ _ _ _ _ w4253 _ _ _ _]
              tunnel: w3841 -> [_ _ _ _ _ _ w4333 _ _ _]
              tunnel: w3840 -> [_ _ _ _ _ _ _ w4413 _ _]
              tunnel: w3839 -> [_ _ _ _ _ _ _ _ w4493 _]
              tunnel: w3838 -> [_ _ _ _ _ _ _ _ _ w4573]
              tunnel: w3835 -> [w3856 w3937 w4017 w4097 w4177 w4257 w4337 w4417 w4497 w4577]
              tunnel: w3834 -> [w3855 w3936 w4016 w4096 w4176 w4256 w4336 w4416 w4496 w4576]
              tunnel: w3833 -> [w3854 w3935 w4015 w4095 w4175 w4255 w4335 w4415 w4495 w4575]
              tunnel: w3832 -> [w3853 w3934 w4014 w4094 w4174 w4254 w4334 w4414 w4494 w4574]
              frame #0 {
                n2160 = case shown="True" w3857 {
                  tunnel: w3856 -> [_ w3862]
                  tunnel: w3855 -> [_ w3861]
                  tunnel: w3854 -> [_ w3859]
                  tunnel: w3853 -> [_ w3858]
                  frame False {
                  }
                  frame True {
                    n2161 = local read "DISP LAB01-1"() -> (w3863:T4)
                    n2162 = local read "SIG LAB01-1"() -> (w3864:T2)
                    n2163 = local read "ON L01-1"() -> (w3860:cluster{"amps":dbl, "volts":dbl, "pf":dbl})
                    n2164 = Unbundle(w3864) -> ("AMPS"=w3870:dbl, "VOLTS"=w3868:dbl, "PF"=w3867:dbl, "Tmp Live"=w3866:dbl, "Tmp Neut"=w3869:dbl)
                    n2165 = Unbundle(w3863) -> ("CYCLE"=w3865:dbl)  [unwired: 2 out]
                    n2166 = stacked-sequence {
                      tunnel: w3870 -> [w3874 w3893]
                      tunnel: w3869 -> [_ w3892]
                      tunnel: w3868 -> [w3873 w3891]
                      tunnel: w3867 -> [w3872 w3890]
                      tunnel: w3866 -> [_ w3889]
                      tunnel: w3865 -> [_ w3888]
                      tunnel: w3862 -> [_ w3887]
                      tunnel: w3861 -> [w3875 _]
                      tunnel: w3860 -> [w3871 w3885]
                      tunnel: w3859 -> [_ w3886]
                      tunnel: w3858 -> [_ w3881]
                      frame #0 {
                        n2167 = case shown="True" w3875 {
                          tunnel: w3874 -> [_ w3880]
                          tunnel: w3873 -> [_ w3879]
                          tunnel: w3872 -> [_ w3878]
                          tunnel: w3871 -> [_ w3876]
                          frame False {
                          }
                          frame True {
                            n2168 = Bundle(cluster=w3876, "amps"=w3880, "volts"=w3879, "pf"=w3878) -> (w3877:cluster{"amps":dbl, "volts":dbl, "pf":dbl})
                            n2169 = local write "ON L01-1"(w3877) -> ()
                          }
                        }
                      }
                      frame #1 {
                        n2170 = Unbundle(w3885) -> ("amps"=w3884:dbl, "volts"=w3883:dbl, "pf"=w3882:dbl)
                        n2171 = case shown="True" w3886 {
                          tunnel: w3893 -> [_ w3894]
                          tunnel: w3892 -> [_ w3932]
                          tunnel: w3891 -> [_ _]
                          tunnel: w3890 -> [_ _]
                          tunnel: w3889 -> [_ w3931]
                          tunnel: w3888 -> [_ w3930]
                          tunnel: w3887 -> [_ w3898]
                          tunnel: w3884 -> [_ w3895]
                          tunnel: w3883 -> [_ w3927]
                          tunnel: w3882 -> [_ w3926]
                          tunnel: w3881 -> [_ w3896]
                          frame False {
                          }
                          frame True {
                            n2172 = local read "TDMS LAB01-1"() -> (w3929:refnum<k34>)
                            n2173 = Build Array(w3927) -> (w3923:dbl[])
                            n2174 = Build Array(w3926) -> (w3922:dbl[])
                            n2175 = Build Array(w3931) -> (w3921:dbl[])
                            n2176 = Build Array(w3932) -> (w3920:dbl[])
                            n2177 = Build Array(w3895) -> (w3925:dbl[])
                            n2178 = Build Array(w3894) -> (w3924:dbl[])
                            n2179 = Build Array(w3930) -> (w3919:dbl[])
                            n2180 = Build Array("AMPS ON", "AMPS OFF", "VOLTS", "PF", "TEMP Live", "TEMP Neut", "CYCLE") -> (w3903:string[])
                            n2181 = Bundle By Name("Y"=w3925, "t0"=w3896) -> (w3918:waveform(dbl))  [unwired: 1 in]
                            n2182 = Bundle By Name("Y"=w3924, "t0"=w3896) -> (w3917:waveform(dbl))  [unwired: 1 in]
                            n2183 = Bundle By Name("Y"=w3923, "t0"=w3896) -> (w3916:waveform(dbl))  [unwired: 1 in]
                            n2184 = Bundle By Name("Y"=w3922, "t0"=w3896) -> (w3915:waveform(dbl))  [unwired: 1 in]
                            n2185 = Bundle By Name("Y"=w3921, "t0"=w3896) -> (w3914:waveform(dbl))  [unwired: 1 in]
                            n2186 = Bundle By Name("Y"=w3920, "t0"=w3896) -> (w3913:waveform(dbl))  [unwired: 1 in]
                            n2187 = Bundle By Name("Y"=w3919, "t0"=w3896) -> (w3912:waveform(dbl))  [unwired: 1 in]
                            n2188 = Build Array(w3918, w3917, w3916, w3915, w3914, w3913, w3912) -> (w3911:waveform(dbl)[])
                            n2189 = TDMS Write(0:w3929, 5:"TEST VALUES", 7:w3903, 9:w3911) -> (4:w3902:refnum<k34>, 6:w3901:string, 15:w3900:errorcluster)  [unwired: 2 in, 1 out]
                            n2190 = TDMS Write(0:w3902, 5:w3901, 7:"TIME", 9:w3898, 11:w3900) -> (15:w3897:errorcluster)  [unwired: 1 in, 3 out]
                            n2191 = local write "data file error"(w3897) -> ()
                          }
                        }
                      }
                    }
                  }
                }
              }
              frame #1 {
                n2192 = case shown="True" w3933 {
                  tunnel: w3937 -> [_ w3942]
                  tunnel: w3936 -> [_ w3941]
                  tunnel: w3935 -> [_ w3939]
                  tunnel: w3934 -> [_ w3938]
                  frame False {
                  }
                  frame True {
                    n2193 = local read "DISP LAB01-2"() -> (w3943:T4)
                    n2194 = local read "SIG LAB01-2"() -> (w3944:T2)
                    n2195 = local read "ON L01-2"() -> (w3940:cluster{"amps":dbl, "volts":dbl, "pf":dbl})
                    n2196 = Unbundle(w3944) -> ("AMPS"=w3950:dbl, "VOLTS"=w3948:dbl, "PF"=w3947:dbl, "Tmp Live"=w3946:dbl, "Tmp Neut"=w3949:dbl)
                    n2197 = Unbundle(w3943) -> ("CYCLE"=w3945:dbl)  [unwired: 2 out]
                    n2198 = stacked-sequence {
                      tunnel: w3950 -> [w3954 w3973]
                      tunnel: w3949 -> [_ w3972]
                      tunnel: w3948 -> [w3953 w3971]
                      tunnel: w3947 -> [w3952 w3970]
                      tunnel: w3946 -> [_ w3969]
                      tunnel: w3945 -> [_ w3968]
                      tunnel: w3942 -> [_ w3967]
                      tunnel: w3941 -> [w3955 _]
                      tunnel: w3940 -> [w3951 w3965]
                      tunnel: w3939 -> [_ w3966]
